vi "Cleanup.vi"(8 "error in (no error)":errorcluster, 11 "BoardArrayPanel in":refnum<class "BoardArrayPanel.lvclass">) -> (0 "error out":errorcluster)   [LabVIEW 2020, in "PicoG-App.lvlib" / "BoardArrayPanel.lvclass"]
uses:
  BoardArrayPanel.lvclass
  <vilib>/IlluminatedG/IG OOPanel/OOPanel/ArrayPanel/ArrayPanel.lvclass
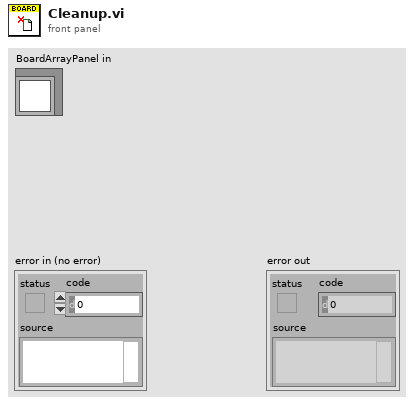
[diagram p1: front panel]
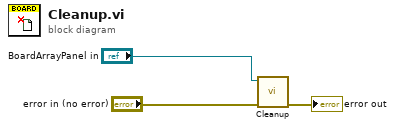
[diagram p0: block diagram]
diagram:
  n1 = call-parent "Cleanup.vi"("error in (no error)"="error in (no error)", "ArrayPanel in"="BoardArrayPanel in") -> ("error out"=→"error out":errorcluster)  [unwired: 9 in]
